vi "dll Install Path.vi"() -> (3 "system directory":path)   [LabVIEW 2018, in "ASIA Pump.lvlib"]
uses:
  ASIA Pump.lvlib
  <vilib>/Utility/sysdir.llb/System Directory Type.ctl
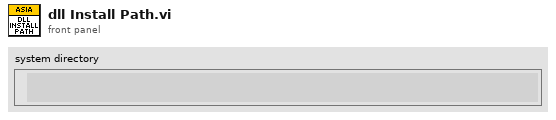
[diagram p1: front panel]
types:
  T1 = typedef "System Directory Type.ctl" = i32
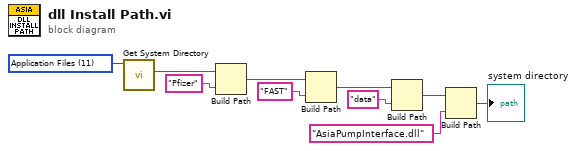
[diagram p0: block diagram]
diagram:
  w1 = T1 11 items=["User Home"=0, "User Desktop"=1, "User Documents"=2, "User Application Data"=3, "User Preferences"=4, "User Temporary"=5, "Public Documents"=6, "Public Application Data"=7, "Public Preferences"=8, "Public Cache"=13, "System Core Libraries"=9, "System Installed Libraries"=10, "Application Files"=11, "Boot Volume Root"=12] ("system directory type")
  n1 = call <vilib>:"Get System Directory.vi"("system directory type"=w1) -> ("system directory"=w2:path)  [unwired: 10 in]
  n2 = Build Path(base path=w2, name or relative path="Pfizer") -> (appended path=w4:path)
  n3 = Build Path(base path=w4, name or relative path="FAST") -> (appended path=w6:path)
  n4 = Build Path(base path=w6, name or relative path="data") -> (appended path=w8:path)
  n5 = Build Path(base path=w8, name or relative path="AsiaPumpInterface.dll") -> (appended path=→"system directory":path)
